vi "5.vi"() -> ()   [LabVIEW 2019]
panel:
  out "RMS":dbl
  out "P-to-P":dbl
  out "+P":dbl
  out "-P":dbl
  out "Waveform Chart":dynamicdata(graph)
  in  "stop (F)":bool
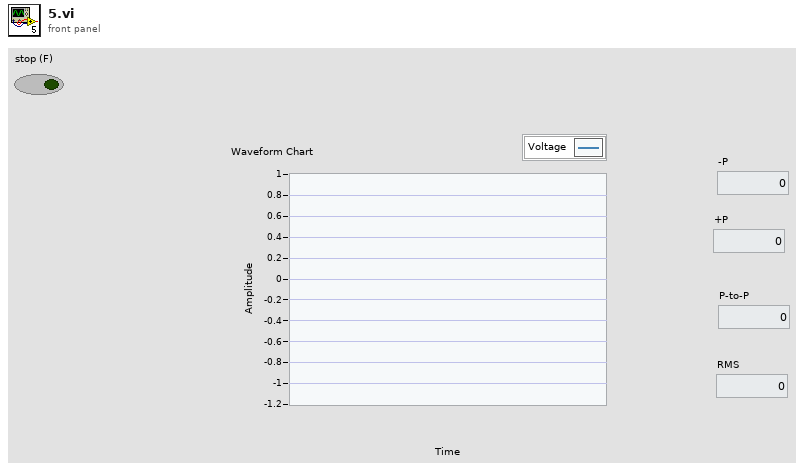
[diagram p1: front panel]
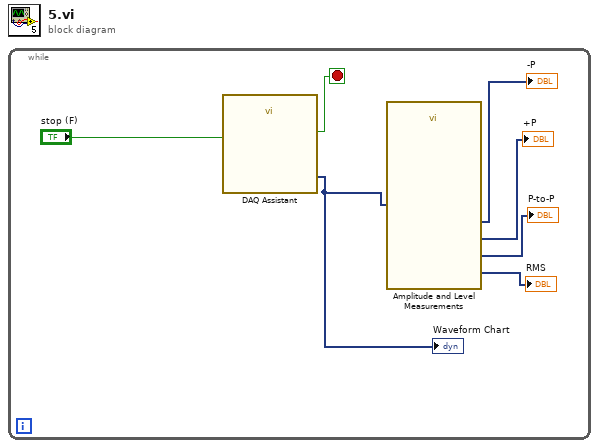
[diagram p0: block diagram]
diagram:
  n1 = while {
    stop <- w6 stop-if-true
    n2 = call "DAQ Assistant"("stop (F)"="stop (F)") -> ("data"=w5:dynamicdata, "stopped"=w6:bool)  [unwired: 15 in, 2 out]
    "Waveform Chart" <- w5
    n3 = call "Amplitude and Level Measurements"("Signals"=w5) -> ("RMS"=→"RMS":dynamicdata, "Negative Peak"=→"-P":dynamicdata, "Positive Peak"=→"P-to-P":dynamicdata, "Peak to Peak"=→"+P":dynamicdata)  [unwired: 10 in, 1 out]
  }
